vi "Main Host v3.vi"() -> ()   [LabVIEW 2018]
uses:
  Target Lossy Data.ctl
  Sensor Data.ctl
  Messages.ctl
  <vilib>/Utility/Variable/NI_VariableUtilities.lvlib
panel:
  in  "Gain":dbl=86.7
  in  "Use phi Remainder?":bool
  out "Right Foot Loaded?":bool
  out "Left Foot Loaded?":bool
  in  "Phi_end":dbl=2.0
  in  "Phi_1":dbl
  in  "Logging Duration (s)":dbl=30.0
  in  "Data Filename":string="cp_test"
  out "error out":errorcluster
  in  "Bias Current (A)":dbl=1.0
  in  "F Threshold":u32=400
  in  "d_F Threshold":u32=5
  in  "Tab Control":enum32{"Controls", "Plots", "Force Plots"}(tab)
  in  "Escon P":dbl
  in  "Escon I":dbl
  in  "N":u32=3
  in  "Benchtop Test?":bool
  in  "mV / N":dbl=2.2485
  in  "Use Simulation Data?":bool
  in  "# PCA Samples":u16=10000
  in  "# UART Bytes":u8=22
  in  "Logging Mode":bool
  in  "Prosthetic Side":bool=TRUE
  out "Time":string
  out "Date":string
  in  "Period [microseconds]":u32=2000
  in  "Max Current Rate (A)":dbl=0.5
  in  "Escon Max Current":dbl=14.0
  in  "Cutoff Freq [Hz]":dbl=50.0
  out "Motor Current":T1(graph)
  out "Ankle Kinematics":T2(graph)
  out "Ankle Torques":T3(graph)
  out "Has Index Pulse \nOccurred yet?":bool
  out "Phase":T4(graph)
  out "Gait %":T4(graph)
  out "IMU Readings":T5(graph)
  out "Right Heel Strike FSM":u32(graph)
  out "Right Force Rate":cluster{"d_GRF R":dbl, "dF_th":dbl, dbl}(graph)
  out "Left Force Rate":cluster{"d_GRF L":dbl, "dF_th":dbl, dbl}(graph)
  out "Left Heel Strike FSM":u32(graph)
  out "Right Force":cluster{"GRF R":dbl, "GRF R":dbl, "F_th":dbl}(graph)
  out "Left Force":cluster{"GRF L":dbl, "GRF L":dbl, "F_th":dbl}(graph)
  in  "Control Gain":dbl(knob) scale=0.0..1.0
  out "Target Lossy Data":T6
  out "Currently Logging Data":bool
  in  "Log data":bool
  in  "Activate Controller":bool
  in  "Stop":bool
  # "x pi"
  # "x pi"
  # "No\nFalse"
  # "Yes\nTrue"
  # "Button"
  # "Vicon"
  # "Raw IMU: 20\nKalman: 22"
  # "Left\nFalse"
  # "Right\nTrue"
  # "(2 = heel contact, 1 = no heel contact)"
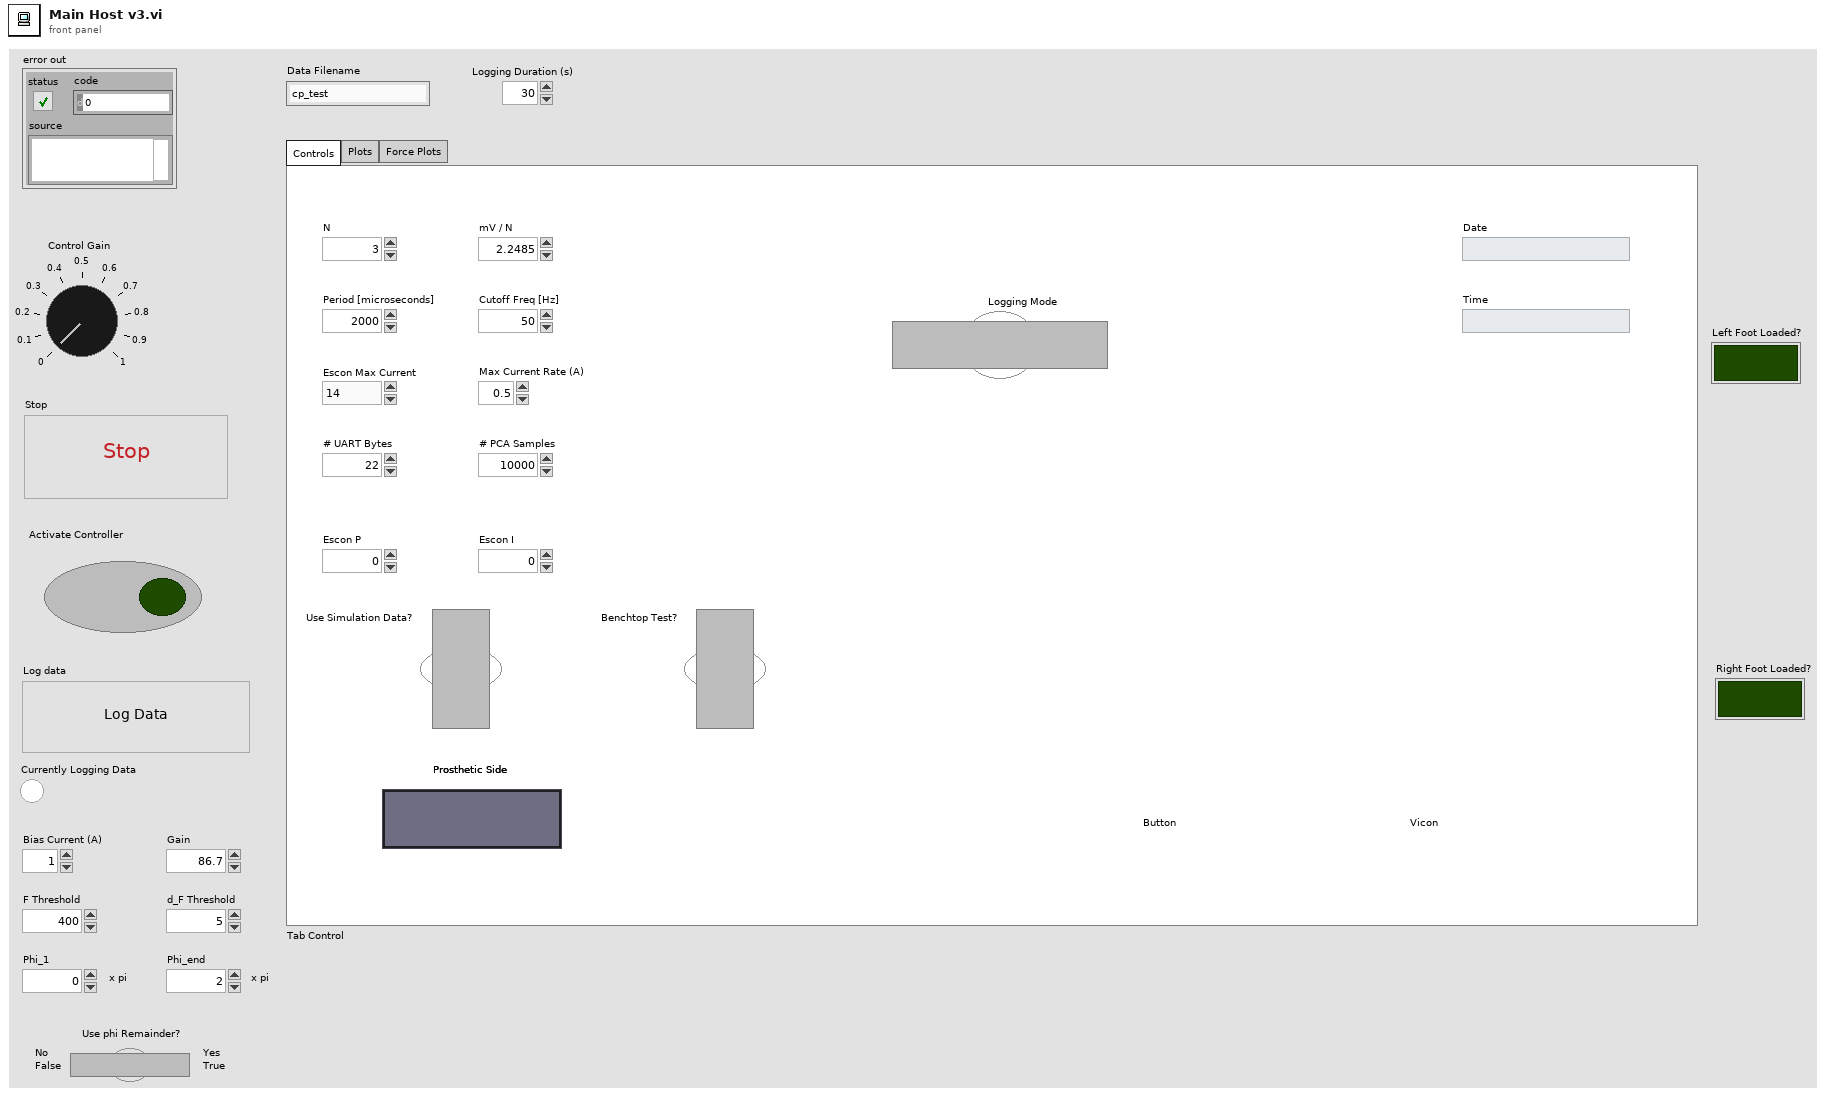
[diagram p1: front panel]
types:
  T1 = cluster{"Motor Command":dbl, "Motor Current":dbl}
  T2 = cluster{"Desired Ankle Traj.":dbl, "Ankle Encoder Angle":dbl}
  T3 = cluster{"Torque Reference":dbl, "Passive Torque":dbl}
  T4 = cluster{"Phase Variable":dbl, "Phase Variable":dbl}
  T5 = cluster{"Roll":dbl, "Pitch":dbl, "Thigh Angle":dbl, "Roll":dbl, "Pitch":dbl, "Thigh Angle":dbl}
  T6 = typedef "Target Lossy Data.ctl" = cluster{"Active Controller":bool, "Log Trigger":bool, "Sensors":T7, "Motor Command":dbl, "Phase Variable":dbl, "Left HS State":u32, "Left Heel Strike Pulse":bool, "Gait %":dbl, "Torque Reference":dbl, "Passive Torque":dbl, "F_th":dbl, "dF_th":dbl, "d_GRF L":dbl, "GRF L":dbl, "Transmission Ratio":dbl, "Desired Ankle Traj.":dbl, "Right HS State":u32, "Right Heel Strike Pulse":bool, "d_GRF R":dbl, "GRF R":dbl}
  T7 = typedef "Sensor Data.ctl" = cluster{"Motor Current":dbl, "Motor Velocity":dbl, "Ankle Encoder Angle":dbl, "GRF L":dbl, "GRF R":dbl, "Index pulse?":bool, "Roll":dbl, "Pitch":dbl, "Yaw":dbl, "Thigh Angle":dbl}
  T8 = typedef "Messages.ctl" = enum16{"Stop", "Activate/Deactivate Controller", "Log Data", "FF Control Gain Change", "F Thr Change", "dF Thr Change", "Bias Current Change", "Filename Change", "Logging Duration Change", "Phi 1 Change", "Phi End Change", "Phi Remainder Change", "Cutoff Freq Changed", "Control Gain Changed", "Num Phi Param Samples Changed"}
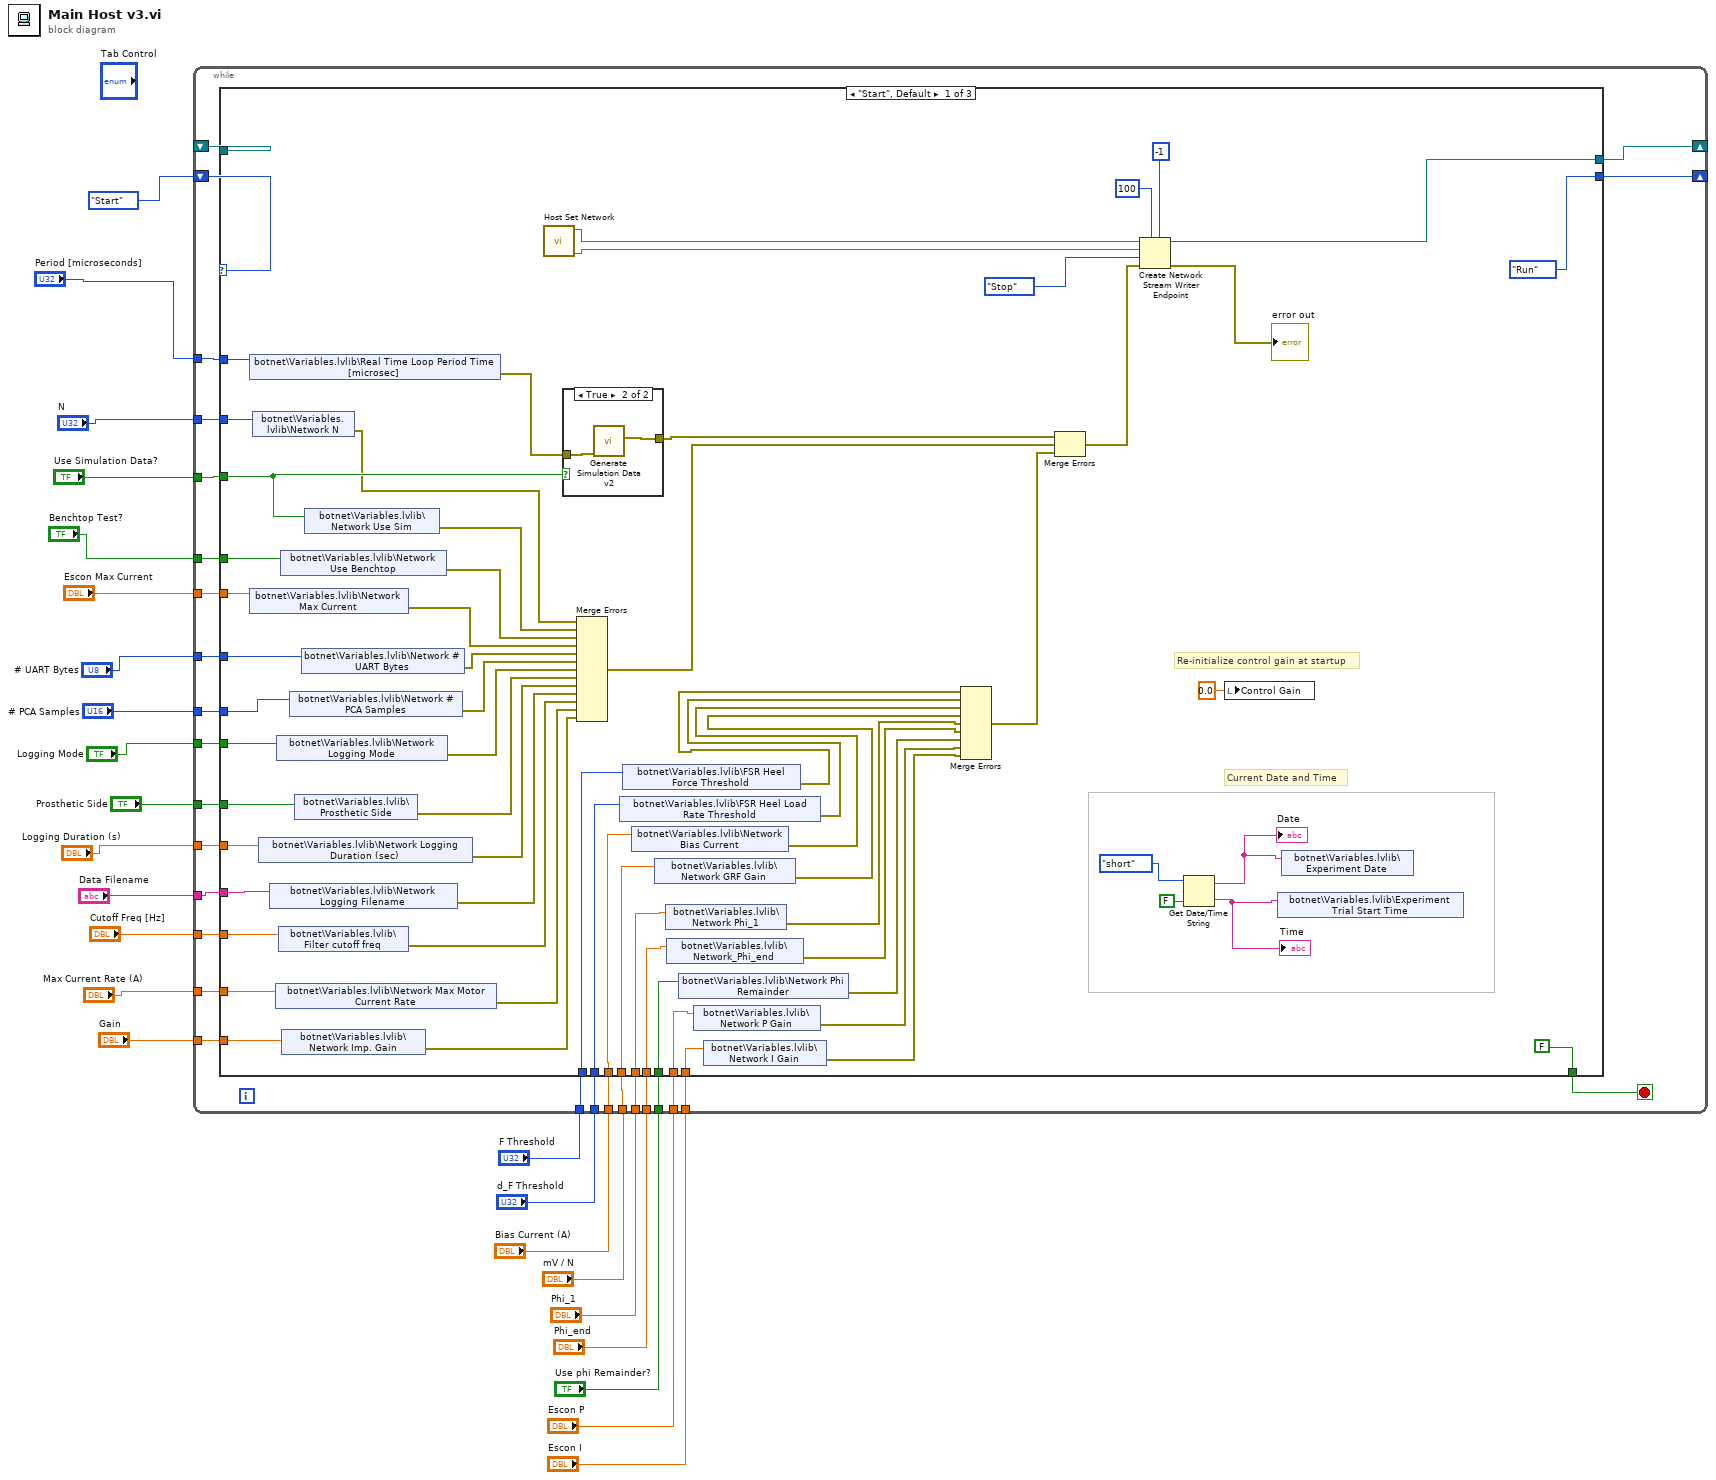
[diagram p0: block diagram]
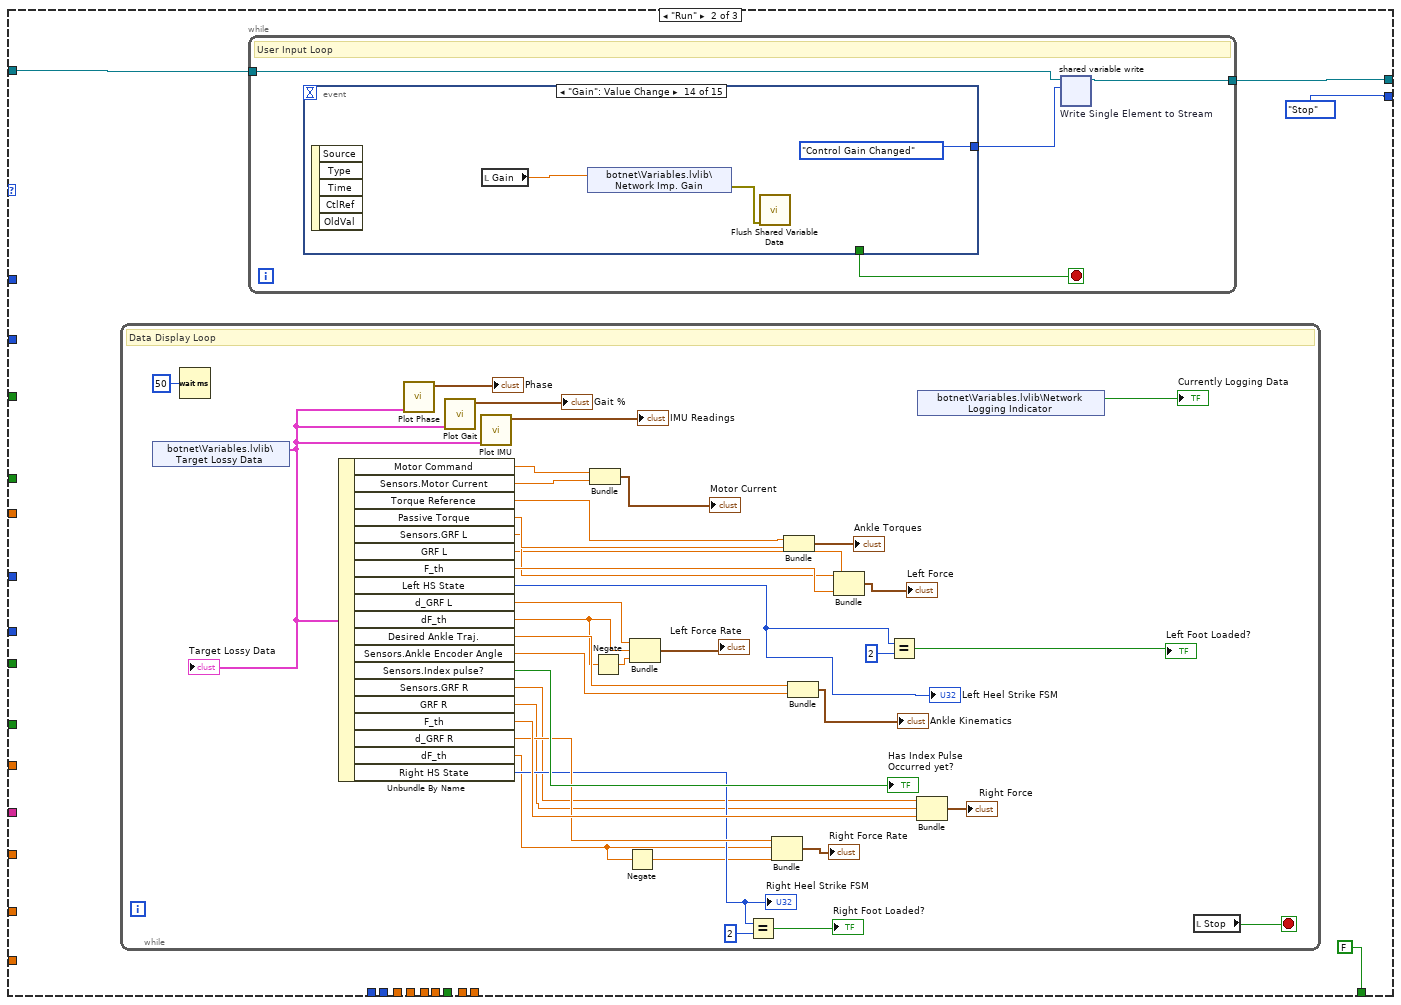
[diagram p3: hidden frame]
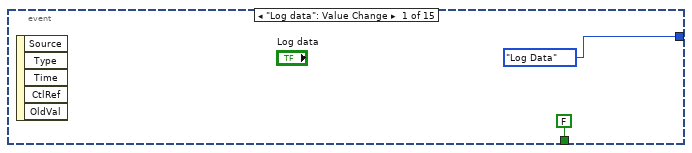
[diagram p4: hidden frame]
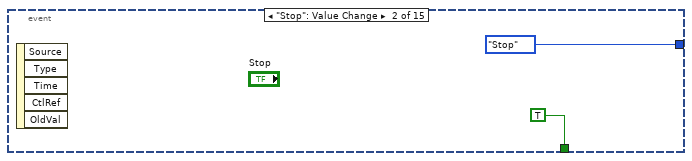
[diagram p5: hidden frame]
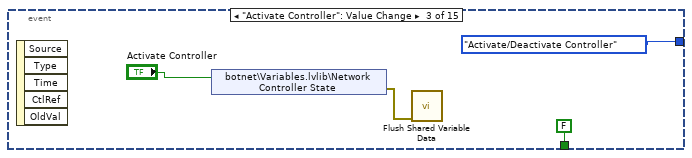
[diagram p6: hidden frame]
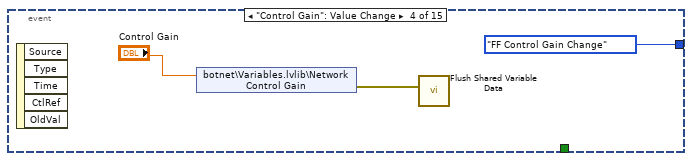
[diagram p7: hidden frame]
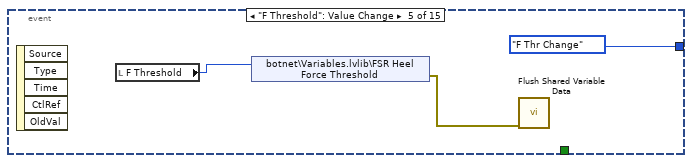
[diagram p8: hidden frame]
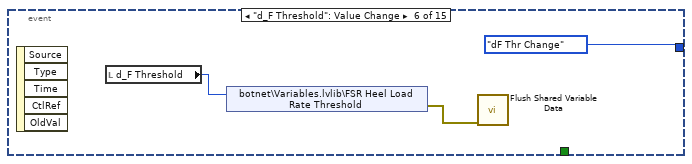
[diagram p9: hidden frame]
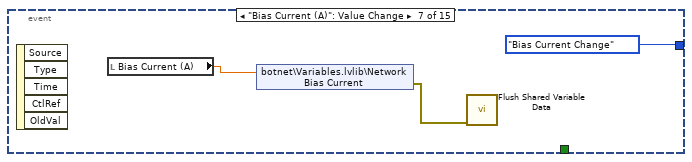
[diagram p10: hidden frame]
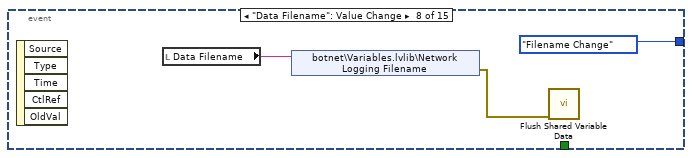
[diagram p11: hidden frame]
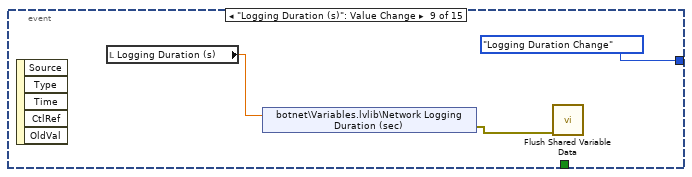
[diagram p12: hidden frame]
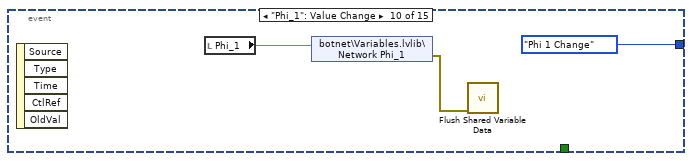
[diagram p13: hidden frame]
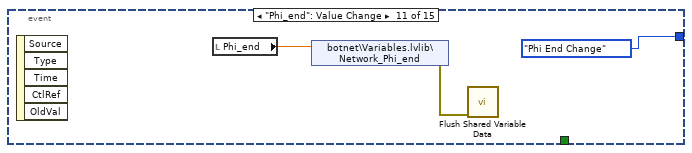
[diagram p14: hidden frame]
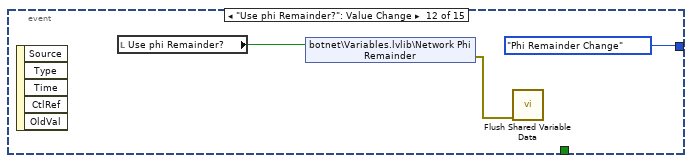
[diagram p15: hidden frame]
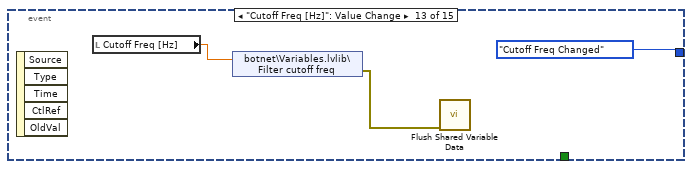
[diagram p16: hidden frame]
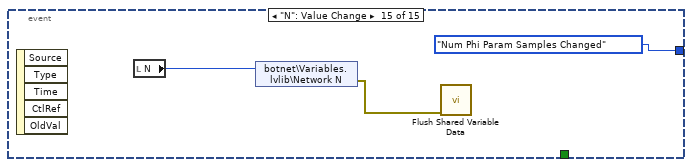
[diagram p17: hidden frame]
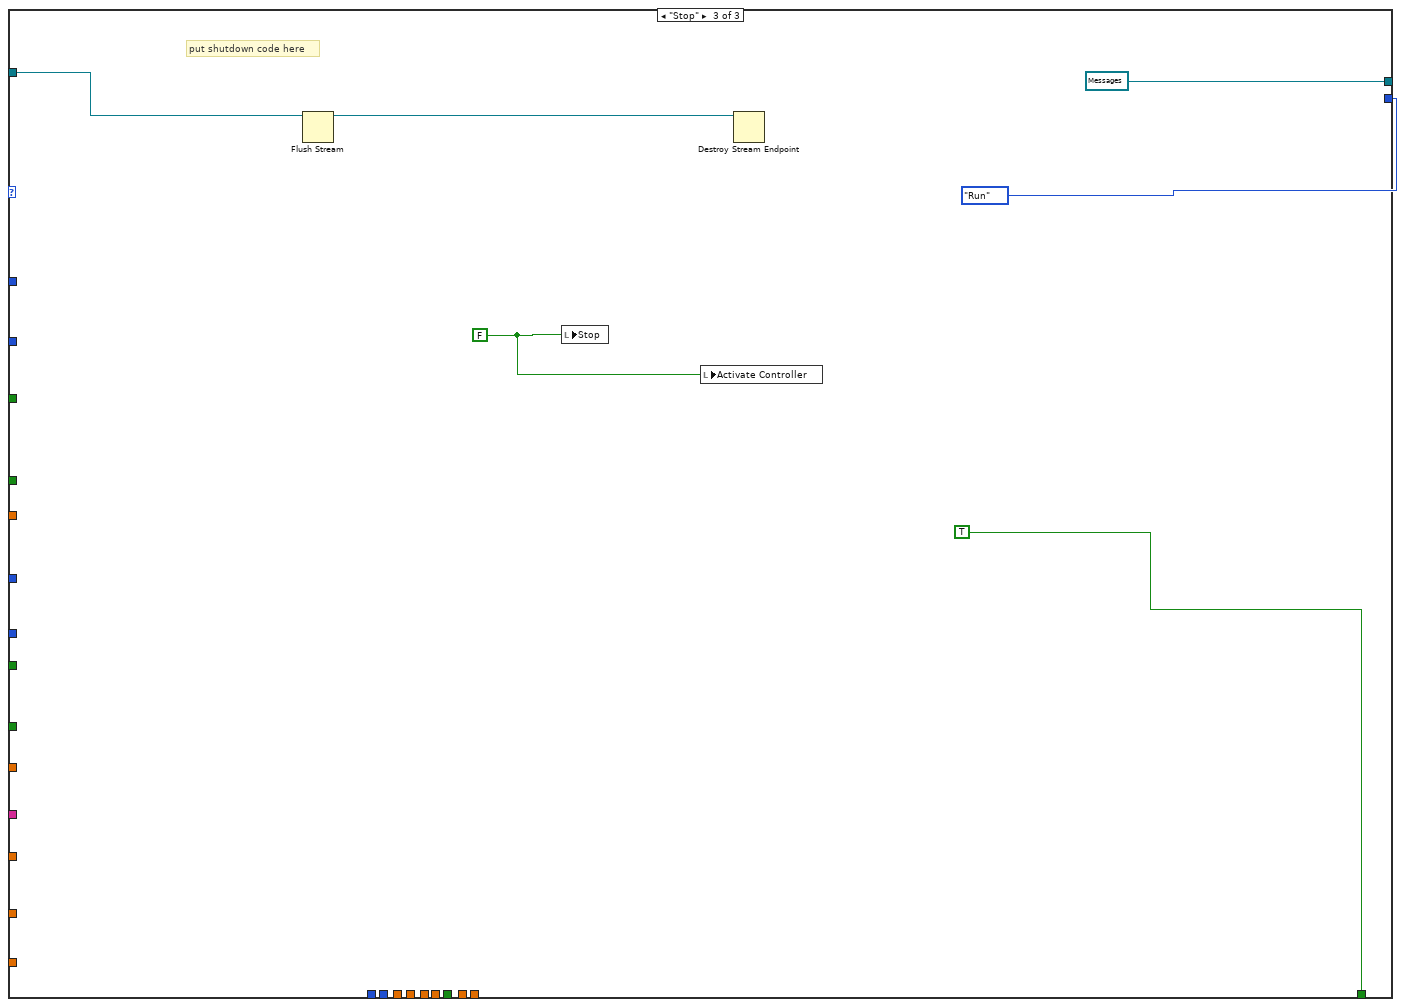
[diagram p18: hidden frame]
diagram:
  n1 = while {
    shift-right: [w52] -> _
    shift-left: enum16{"Start", "Run", "Stop"}."Start" -> [w51]
    shift-right: [w49] -> _
    shift-left: _ -> [w48]
    tunnel: "Period [microseconds]" -> [w47]
    tunnel: "Logging Duration (s)" -> [w46]
    tunnel: "Data Filename" -> [w45]
    tunnel: "Max Current Rate (A)" -> [w44]
    tunnel: "Gain" -> [w43]
    tunnel: "Prosthetic Side" -> [w42]
    tunnel: "Cutoff Freq [Hz]" -> [w41]
    tunnel: "Logging Mode" -> [w40]
    tunnel: "Use Simulation Data?" -> [w39]
    tunnel: "# UART Bytes" -> [w38]
    tunnel: "# PCA Samples" -> [w37]
    tunnel: "F Threshold" -> [w36]
    tunnel: "d_F Threshold" -> [w35]
    tunnel: "Bias Current (A)" -> [w34]
    tunnel: "Escon Max Current" -> [w33]
    tunnel: "mV / N" -> [w32]
    tunnel: "Phi_1" -> [w31]
    tunnel: "Phi_end" -> [w30]
    tunnel: "Use phi Remainder?" -> [w29]
    tunnel: "Benchtop Test?" -> [w28]
    tunnel: "N" -> [w27]
    tunnel: "Escon P" -> [w26]
    tunnel: "Escon I" -> [w25]
    stop <- w50 stop-if-true
    n2 = case shown="\"Start\", Default" w51 {
      tunnel: [enum16{"Start", "Run", "Stop"}."Run" enum16{"Start", "Run", "Stop"}."Stop" enum16{"Start", "Run", "Stop"}."Run"] -> w52
      tunnel: [FALSE FALSE TRUE] -> w50
      tunnel: [w112 w120 w212] -> w49
      tunnel: w48 -> [_ w121 w214]
      tunnel: w47 -> [w111 _ _]
      tunnel: w46 -> [w71 _ _]
      tunnel: w45 -> [w109 _ _]
      tunnel: w44 -> [w108 _ _]
      tunnel: w43 -> [w107 _ _]
      tunnel: w42 -> [w103 _ _]
      tunnel: w41 -> [w100 _ _]
      tunnel: w40 -> [w97 _ _]
      tunnel: w39 -> [w96 _ _]
      tunnel: w38 -> [w95 _ _]
      tunnel: w37 -> [w94 _ _]
      tunnel: w36 -> [w82 _ _]
      tunnel: w35 -> [w81 _ _]
      tunnel: w34 -> [w80 _ _]
      tunnel: w33 -> [w74 _ _]
      tunnel: w32 -> [w73 _ _]
      tunnel: w31 -> [w69 _ _]
      tunnel: w30 -> [w68 _ _]
      tunnel: w29 -> [w65 _ _]
      tunnel: w28 -> [w62 _ _]
      tunnel: w27 -> [w58 _ _]
      tunnel: w26 -> [w56 _ _]
      tunnel: w25 -> [w55 _ _]
      frame "Start", Default {
        # "Current Date and Time"
        # "Re-initialize control gain at startup"
        n3 = shared-variable "botnet\\Variables.lvlib\\Real Time Loop Period Time [microsec]"(w111) -> (error out=w110:errorcluster)  [unwired: 1 in]
        n4 = shared-variable "botnet\\Variables.lvlib\\Network Max Current"(w74) -> (error out=w75:errorcluster)  [unwired: 1 in]
        n5 = shared-variable "botnet\\Variables.lvlib\\Network N"(w58) -> (error out=w57:errorcluster)  [unwired: 1 in]
        n6 = shared-variable "botnet\\Variables.lvlib\\Network Logging Duration (sec)"(w71) -> (error out=w70:errorcluster)  [unwired: 1 in]
        n7 = shared-variable "botnet\\Variables.lvlib\\Network Logging Filename"(w109) -> (error out=w87:errorcluster)  [unwired: 1 in]
        n8 = shared-variable "botnet\\Variables.lvlib\\Network Max Motor Current Rate"(w108) -> (error out=w85:errorcluster)  [unwired: 1 in]
        n9 = shared-variable "botnet\\Variables.lvlib\\Network Logging Mode"(w97) -> (error out=w89:errorcluster)  [unwired: 1 in]
        n10 = shared-variable "botnet\\Variables.lvlib\\Filter cutoff freq"(w100) -> (error out=w86:errorcluster)  [unwired: 1 in]
        n11 = shared-variable "botnet\\Variables.lvlib\\Network Use Benchtop"(w62) -> (error out=w61:errorcluster)  [unwired: 1 in]
        n12 = shared-variable "botnet\\Variables.lvlib\\Network Imp. Gain"(w107) -> (error out=w84:errorcluster)  [unwired: 1 in]
        n13 = shared-variable "botnet\\Variables.lvlib\\Network # PCA Samples"(w94) -> (error out=w90:errorcluster)  [unwired: 1 in]
        n14 = shared-variable "botnet\\Variables.lvlib\\Prosthetic Side"(w103) -> (error out=w88:errorcluster)  [unwired: 1 in]
        n15 = shared-variable "botnet\\Variables.lvlib\\Network # UART Bytes"(w95) -> (error out=w91:errorcluster)  [unwired: 1 in]
        n16 = shared-variable "botnet\\Variables.lvlib\\Network Use Sim"(w96) -> (error out=w63:errorcluster)  [unwired: 1 in]
        n17 = call "Host Set Network.vi"() -> ("Reader"=w59:string, "Writer"=w60:string)  [unwired: 10 in]
        n18 = case shown="True" w96 {
          tunnel: [w117 w119] -> w93
          tunnel: w110 -> [w117 w118]
          frame False {
          }
          frame True {
            n19 = call "Generate Simulation Data v2.vi"("error in (no error)"=w118) -> ("Error Out"=w119:errorcluster)  [unwired: 10 in]
          }
        }
        n20 = Merge Errors(w57, w63, w61, w75, w91, w90, w89, w88, w70, w87, w86, w85, w84) -> (w83:errorcluster)
        n21 = shared-variable "botnet\\Variables.lvlib\\FSR Heel Load Rate Threshold"(w81) -> (error out=w77:errorcluster)  [unwired: 1 in]
        n22 = shared-variable "botnet\\Variables.lvlib\\FSR Heel Force Threshold"(w82) -> (error out=w76:errorcluster)  [unwired: 1 in]
        n23 = shared-variable "botnet\\Variables.lvlib\\Network Bias Current"(w80) -> (error out=w78:errorcluster)  [unwired: 1 in]
        n24 = shared-variable "botnet\\Variables.lvlib\\Network GRF Gain"(w73) -> (error out=w72:errorcluster)  [unwired: 1 in]
        n25 = shared-variable "botnet\\Variables.lvlib\\Network Phi_1"(w69) -> (error out=w67:errorcluster)  [unwired: 1 in]
        n26 = shared-variable "botnet\\Variables.lvlib\\Network_Phi_end"(w68) -> (error out=w66:errorcluster)  [unwired: 1 in]
        n27 = shared-variable "botnet\\Variables.lvlib\\Network Phi Remainder"(w65) -> (error out=w64:errorcluster)  [unwired: 1 in]
        n28 = shared-variable "botnet\\Variables.lvlib\\Network P Gain"(w56) -> (error out=w54:errorcluster)  [unwired: 1 in]
        n29 = shared-variable "botnet\\Variables.lvlib\\Network I Gain"(w55) -> (error out=w53:errorcluster)  [unwired: 1 in]
        n30 = Merge Errors(w76, w77, w78, w72, w67, w66, w64, w54, w53) -> (w79:errorcluster)
        n31 = Merge Errors(w93, w83, w79) -> (w92:errorcluster)
        n32 = Create Network Stream Writer Endpoint(5:-1 ("timeout in ms (-1)"), 7:100 ("writer buffer size"), 8:w92, 9:Messages."Stop" ("Messages"), 10:w59, 11:w60) -> (0:→"error out":errorcluster, 3:w112:refnum<k21>)  [unwired: 1 in]
        n33 = Get Date/Time String(date format (0)=enum16{"short", "long", "abbreviated"}."short", want seconds? (F)=FALSE) -> (date string=w102:string, time string=w101:string)  [unwired: 1 in]
        "Date" <- w102
        "Time" <- w101
        n34 = local write "Control Gain"(0.0 ("Control Gain")) -> ()
        n35 = shared-variable "botnet\\Variables.lvlib\\Experiment Trial Start Time"(w101) -> ()  [unwired: 1 in, 1 out]
        n36 = shared-variable "botnet\\Variables.lvlib\\Experiment Date"(w102) -> ()  [unwired: 1 in, 1 out]
      }
      frame "Run" {
        n37 = while {
          stop <- w161 stop-if-true
          # "Data Display Loop"
          n38 = shared-variable "botnet\\Variables.lvlib\\Target Lossy Data"() -> (w125:T6)  [unwired: 1 in, 1 out]
          "Target Lossy Data" <- w125
          n39 = Wait (ms)(milliseconds to wait=u32 50) -> ()  [unwired: 1 out]
          n40 = Unbundle By Name(w125) -> ("Motor Command"=w154:dbl, "Sensors.Motor Current"=w153:dbl, "Torque Reference"=w150:dbl, "Passive Torque"=w149:dbl, "Sensors.GRF L"=w135:dbl, "GRF L"=w134:dbl, "F_th"=w136:dbl, "Left HS State"=w137:u32, "d_GRF L"=w160:dbl, "dF_th"=w131:dbl, "Desired Ankle Traj."=w156:dbl, "Sensors.Ankle Encoder Angle"=w124:dbl, "Sensors.Index pulse?"=→"Has Index Pulse \nOccurred yet?":bool, "Sensors.GRF R"=w139:dbl, "GRF R"=w138:dbl, "F_th"=w147:dbl, "d_GRF R"=w143:dbl, "dF_th"=w129:dbl, "Right HS State"=w140:u32)
          "Left Heel Strike FSM" <- w137
          "Right Heel Strike FSM" <- w140
          n41 = call "Plot Phase.vi"("Target Lossy Data"=w125) -> ("Phase Waveform"=→"Phase":T4)  [unwired: 10 in]
          n42 = call "Plot Gait.vi"("Target Lossy Data"=w125) -> ("Gait % Waveform"=→"Gait %":T4)  [unwired: 10 in]
          n43 = call "Plot IMU.vi"("Target Lossy Data"=w125) -> ("IMU Waveform"=→"IMU Readings":T5)  [unwired: 10 in]
          n44 = Bundle("Motor Command"=w154, "Motor Current"=w153) -> (→"Motor Current":T1)  [unwired: 1 in]
          n45 = Negate(x=w131) -> (-x=w132:dbl)
          n46 = Negate(x=w129) -> (-x=w130:dbl)
          n47 = Bundle("d_GRF L"=w160, "dF_th"=w131, w132) -> (→"Left Force Rate":cluster{"d_GRF L":dbl, "dF_th":dbl, dbl})  [unwired: 1 in]
          n48 = Equal?(x=w140, y=u32 2) -> (x = y?=→"Right Foot Loaded?":bool)
          n49 = Bundle("d_GRF R"=w143, "dF_th"=w129, w130) -> (→"Right Force Rate":cluster{"d_GRF R":dbl, "dF_th":dbl, dbl})  [unwired: 1 in]
          n50 = Bundle("Torque Reference"=w150, "Passive Torque"=w149) -> (→"Ankle Torques":T3)  [unwired: 1 in]
          n51 = Bundle("Desired Ankle Traj."=w156, "Ankle Encoder Angle"=w124) -> (→"Ankle Kinematics":T2)  [unwired: 1 in]
          n52 = Bundle("GRF L"=w135, "GRF L"=w134, "F_th"=w136) -> (→"Left Force":cluster{"GRF L":dbl, "GRF L":dbl, "F_th":dbl})  [unwired: 1 in]
          n53 = Equal?(x=w137, y=u32 2) -> (x = y?=→"Left Foot Loaded?":bool)
          n54 = Bundle("GRF R"=w139, "GRF R"=w138, "F_th"=w147) -> (→"Right Force":cluster{"GRF R":dbl, "GRF R":dbl, "F_th":dbl})  [unwired: 1 in]
          n55 = shared-variable "botnet\\Variables.lvlib\\Network Logging Indicator"() -> (→"Currently Logging Data":bool)  [unwired: 1 in, 1 out]
          n56 = local read "Stop"() -> (w161:bool)
        }
        n57 = while {
          tunnel: w121 -> [w165]
          tunnel: [w164] -> w120
          stop <- w166 stop-if-true
          # "User Input Loop"
          n58 = event shown="[13] \"Gain\": Value Change" {
            selector: _ -> [_ _ _ _ _ _ _ _ _ _ _ _ _ _ _]
            dyn-events: _ -> [_ _ _ _ _ _ _ _ _ _ _ _ _ _ _]
            timeout: _ -> [_ _ _ _ _ _ _ _ _ _ _ _ _ _ _]
            tunnel: [FALSE TRUE FALSE _ _ _ _ _ _ _ _ _ _ _ _] -> w166
            tunnel: [Messages."Log Data" ("Messages") Messages."Stop" ("Messages") Messages."Activate/Deactivate Controller" ("Messages") Messages."FF Control Gain Change" ("Messages") Messages."F Thr Change" ("Messages") Messages."dF Thr Change" ("Messages") Messages."Bias Current Change" ("Messages") Messages."Filename Change" ("Messages") Messages."Logging Duration Change" ("Messages") Messages."Phi 1 Change" ("Messages") Messages."Phi End Change" ("Messages") Messages."Phi Remainder Change" ("Messages") Messages."Cutoff Freq Changed" ("Messages") Messages."Control Gain Changed" ("Messages") Messages."Num Phi Param Samples Changed" ("Messages")] -> w163
            event "Log data": Value Change {
              n59 = event-data() -> ()  [unwired: 1 in, 5 out]
            }
            event "Stop": Value Change {
              n60 = event-data() -> ()  [unwired: 1 in, 5 out]
            }
            event "Activate Controller": Value Change {
              n61 = event-data() -> ()  [unwired: 1 in, 5 out]
              n62 = shared-variable "botnet\\Variables.lvlib\\Network Controller State"("Activate Controller") -> (error out=w171:errorcluster)  [unwired: 1 in]
              n63 = call <vilib>:"Flush Shared Variable Data.vi"("error in (no error)"=w171) -> ()  [unwired: 10 in, 1 out]
            }
            event "Control Gain": Value Change {
              n64 = event-data() -> ()  [unwired: 1 in, 5 out]
              n65 = shared-variable "botnet\\Variables.lvlib\\Network Control Gain"("Control Gain") -> (error out=w176:errorcluster)  [unwired: 1 in]
              n66 = call <vilib>:"Flush Shared Variable Data.vi"("error in (no error)"=w176) -> ()  [unwired: 10 in, 1 out]
            }
            event "F Threshold": Value Change {
              n67 = event-data() -> ()  [unwired: 1 in, 5 out]
              n68 = local read "F Threshold"() -> (w178:u32)
              n69 = shared-variable "botnet\\Variables.lvlib\\FSR Heel Force Threshold"(w178) -> (error out=w180:errorcluster)  [unwired: 1 in]
              n70 = call <vilib>:"Flush Shared Variable Data.vi"("error in (no error)"=w180) -> ()  [unwired: 10 in, 1 out]
            }
            event "d_F Threshold": Value Change {
              n71 = event-data() -> ()  [unwired: 1 in, 5 out]
              n72 = local read "d_F Threshold"() -> (w181:u32)
              n73 = shared-variable "botnet\\Variables.lvlib\\FSR Heel Load Rate Threshold"(w181) -> (error out=w183:errorcluster)  [unwired: 1 in]
              n74 = call <vilib>:"Flush Shared Variable Data.vi"("error in (no error)"=w183) -> ()  [unwired: 10 in, 1 out]
            }
            event "Bias Current (A)": Value Change {
              n75 = event-data() -> ()  [unwired: 1 in, 5 out]
              n76 = local read "Bias Current (A)"() -> (w184:dbl)
              n77 = shared-variable "botnet\\Variables.lvlib\\Network Bias Current"(w184) -> (error out=w186:errorcluster)  [unwired: 1 in]
              n78 = call <vilib>:"Flush Shared Variable Data.vi"("error in (no error)"=w186) -> ()  [unwired: 10 in, 1 out]
            }
            event "Data Filename": Value Change {
              n79 = event-data() -> ()  [unwired: 1 in, 5 out]
              n80 = local read "Data Filename"() -> (w189:string)
              n81 = shared-variable "botnet\\Variables.lvlib\\Network Logging Filename"(w189) -> (error out=w188:errorcluster)  [unwired: 1 in]
              n82 = call <vilib>:"Flush Shared Variable Data.vi"("error in (no error)"=w188) -> ()  [unwired: 10 in, 1 out]
            }
            event "Logging Duration (s)": Value Change {
              n83 = event-data() -> ()  [unwired: 1 in, 5 out]
              n84 = local read "Logging Duration (s)"() -> (w191:dbl)
              n85 = shared-variable "botnet\\Variables.lvlib\\Network Logging Duration (sec)"(w191) -> (error out=w190:errorcluster)  [unwired: 1 in]
              n86 = call <vilib>:"Flush Shared Variable Data.vi"("error in (no error)"=w190) -> ()  [unwired: 10 in, 1 out]
            }
            event "Phi_1": Value Change {
              n87 = event-data() -> ()  [unwired: 1 in, 5 out]
              n88 = local read "Phi_1"() -> (w195:dbl)
              n89 = shared-variable "botnet\\Variables.lvlib\\Network Phi_1"(w195) -> (error out=w194:errorcluster)  [unwired: 1 in]
              n90 = call <vilib>:"Flush Shared Variable Data.vi"("error in (no error)"=w194) -> ()  [unwired: 10 in, 1 out]
            }
            event "Phi_end": Value Change {
              n91 = event-data() -> ()  [unwired: 1 in, 5 out]
              n92 = local read "Phi_end"() -> (w197:dbl)
              n93 = shared-variable "botnet\\Variables.lvlib\\Network_Phi_end"(w197) -> (error out=w198:errorcluster)  [unwired: 1 in]
              n94 = call <vilib>:"Flush Shared Variable Data.vi"("error in (no error)"=w198) -> ()  [unwired: 10 in, 1 out]
            }
            event "Use phi Remainder?": Value Change {
              n95 = event-data() -> ()  [unwired: 1 in, 5 out]
              n96 = local read "Use phi Remainder?"() -> (w201:bool)
              n97 = shared-variable "botnet\\Variables.lvlib\\Network Phi Remainder"(w201) -> (error out=w200:errorcluster)  [unwired: 1 in]
              n98 = call <vilib>:"Flush Shared Variable Data.vi"("error in (no error)"=w200) -> ()  [unwired: 10 in, 1 out]
            }
            event "Cutoff Freq [Hz]": Value Change {
              n99 = event-data() -> ()  [unwired: 1 in, 5 out]
              n100 = local read "Cutoff Freq [Hz]"() -> (w203:dbl)
              n101 = shared-variable "botnet\\Variables.lvlib\\Filter cutoff freq"(w203) -> (error out=w202:errorcluster)  [unwired: 1 in]
              n102 = call <vilib>:"Flush Shared Variable Data.vi"("error in (no error)"=w202) -> ()  [unwired: 10 in, 1 out]
            }
            event "Gain": Value Change {
              n103 = event-data() -> ()  [unwired: 1 in, 5 out]
              n104 = local read "Gain"() -> (w207:dbl)
              n105 = shared-variable "botnet\\Variables.lvlib\\Network Imp. Gain"(w207) -> (error out=w206:errorcluster)  [unwired: 1 in]
              n106 = call <vilib>:"Flush Shared Variable Data.vi"("error in (no error)"=w206) -> ()  [unwired: 10 in, 1 out]
            }
            event "N": Value Change {
              n107 = event-data() -> ()  [unwired: 1 in, 5 out]
              n108 = local read "N"() -> (w210:u32)
              n109 = shared-variable "botnet\\Variables.lvlib\\Network N"(w210) -> (error out=w209:errorcluster)  [unwired: 1 in]
              n110 = call <vilib>:"Flush Shared Variable Data.vi"("error in (no error)"=w209) -> ()  [unwired: 10 in, 1 out]
            }
          }
          n111 = shared-variable-write "Write Single Element to Stream"(w165, w163) -> (w164:refnum<k21>)  [unwired: 2 in, 2 out]
        }
      }
      frame "Stop" {
        w212 = refnum<k21> refnum items=["Stop", "Activate/Deactivate Controller", "Log Data", "FF Control Gain Change", "F Thr Change", "dF Thr Change", "Bias Current Change", "Filename Change", "Logging Duration Change", "Phi 1 Change", "Phi End Change", "Phi Remainder Change", "Cutoff Freq Changed", "Control Gain Changed", "Num Phi Param Samples Changed"] ("writer name")
        w211 = FALSE ("Stop")
        # "put shutdown code here"
        n112 = Flush Stream(11:w214) -> (3:w213:refnum<k21>)  [unwired: 3 in, 2 out]
        n113 = local write "Stop"(w211) -> ()
        n114 = local write "Activate Controller"(w211) -> ()
        n115 = Destroy Stream Endpoint(11:w213) -> ()  [unwired: 1 in, 1 out]
      }
    }
  }
